vi "Data Logger (General).vi"(0 "dup path":path, 1 "Numeric":i32, 2 "Text Header":string[][](array[string]), 3 "Data line":string[](array[string]), 4 "file or folder exists?":bool) -> (5 "all rows":string[][](array[string]))   [LabVIEW 2012]
uses:
  <vilib>/Utility/file.llb/Read From Spreadsheet File (string).vi
panel:
  out "dup path 2":path
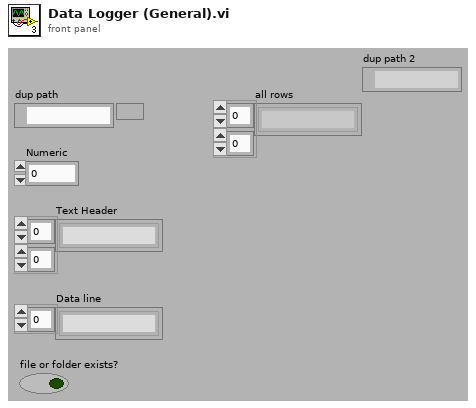
[diagram p1: front panel]
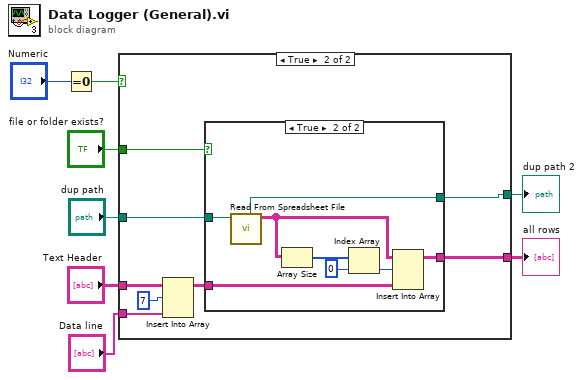
[diagram p0: block diagram]
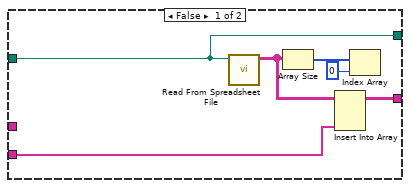
[diagram p2: hidden frame]
diagram:
  n1 = Equal To 0?(x="Numeric") -> (x = 0?=w3:bool)
  n2 = case shown="True" w3 {
    tunnel: "Text Header" -> [_ w22]
    tunnel: "dup path" -> [w9 w16]
    tunnel: [w10 w17] -> w7
    tunnel: "Data line" -> [w11 w20]
    tunnel: "file or folder exists?" -> [_ w19]
    tunnel: [w9 w15] -> w1
    frame False {
      n3 = call-poly <vilib>:"Read From Spreadsheet File.vi"("file path (dialog if empty)"=w9) -> ("all rows"=w12:string[][])  [unwired: 6 in, 4 out]
      n4 = Array Size(array=w12) -> (size(s)=w14:i32[])
      n5 = Insert Into Array(array=w12, new element=w11) -> (w10:string[][])  [unwired: 2 in]
      n6 = Index Array(array=w14, index=0) -> ()  [unwired: 1 out]
    }
    frame True {
      n7 = Insert Into Array(array=w22, index (row)=7, new element=w20) -> (w18:string[][])  [unwired: 1 in]
      n8 = case shown="True" w19 {
        tunnel: w18 -> [w24 w28]
        tunnel: [w24 w26] -> w17
        tunnel: w16 -> [w23 w32]
        tunnel: [w23 w25] -> w15
        frame False {
        }
        frame True {
          n9 = call-poly <vilib>:"Read From Spreadsheet File.vi"("file path (dialog if empty)"=w32) -> ("all rows"=w29:string[][], "new file path (Not A Path if cancelled)"=w25:path)  [unwired: 6 in, 3 out]
          n10 = Array Size(array=w29) -> (size(s)=w31:i32[])
          n11 = Index Array(array=w31, index=0) -> (element=w27:i32)
          n12 = Insert Into Array(array=w29, index (row)=w27, new element=w28) -> (w26:string[][])  [unwired: 1 in]
        }
      }
    }
  }
  "all rows" <- w7
  "dup path 2" <- w1
